vi "Get Lockstep Info.vi"(8 "error in (no error)":errorcluster, 9 "Device Number":string, 10 "Lockstep Group (1)":u8=1, 11 "VISA resource name":refnum<visa-resource-name>) -> (0 "error out":errorcluster, 1 "Axis Offsets":i32[](array[numeric]), 2 "Axis Numbers":i32[](array[numeric]), 3 "VISA resource name out":refnum<visa-resource-name>, 4 "Axis Twists":i32[](array[numeric]))   [LabVIEW 2015, in "Zaber A Series.lvlib"]
doc: "Returns information about a lockstep group. The outputs are:\n- The axis numbers of the axes in the group.\n- The position offsets of each axis relative to the first one, in microsteps.\n- The current twist of each axis relative to the first one.\n\nThis VI requires that the Initialize VI has been called with the same serial port and that the specified lockstep group has been configured."
uses:
  Zaber A Series.lvlib
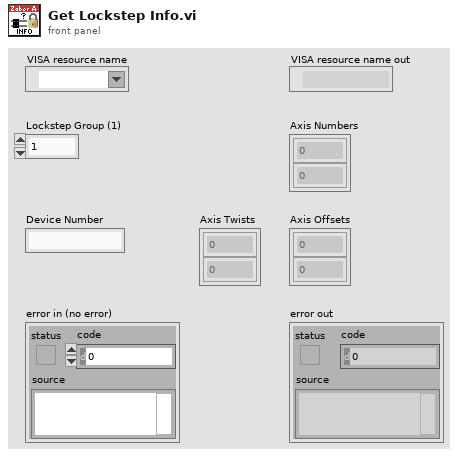
[diagram p1: front panel]
types:
  T1 = cluster{"Device":string, "Axis":string, "Reply Flag":string, "Status":string, "Warning Flags":string, "Data":string}
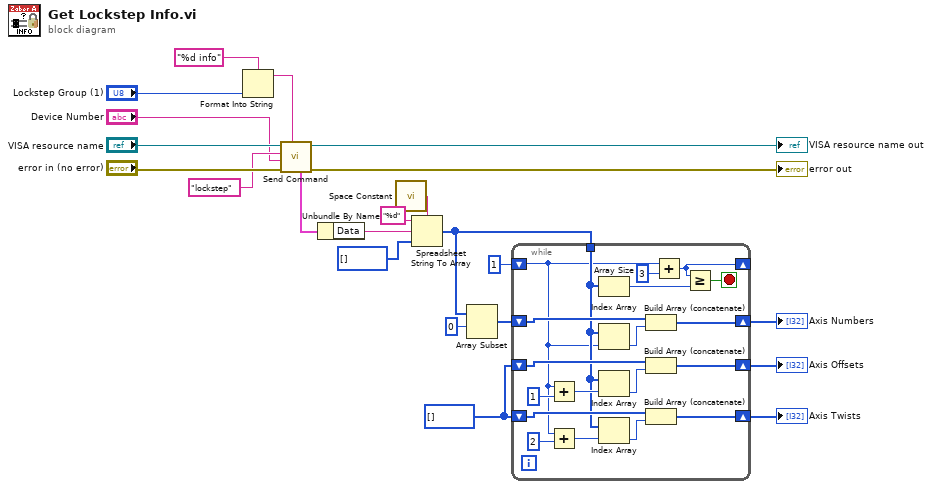
[diagram p0: block diagram]
diagram:
  w2 = i32[] [] ("Axis Offsets")
  n1 = Format Into String(format string="%d info", "Lockstep Group (1)") -> (resulting string=w10:string)  [unwired: 2 in, 1 out]
  n2 = call "Send Command.vi"("Data"=w10, "error in (no error)"="error in (no error)", "Device and Axis"="Device Number", "Command"="lockstep", "VISA resource name"="VISA resource name") -> ("error out"=→"error out":errorcluster, "VISA resource name out"=→"VISA resource name out":refnum<visa-resource-name>, "First Response Bundle"=w9:T1)  [unwired: 1 in, 3 out]
  n3 = Unbundle By Name(w9) -> ("Data"=w19:string)
  n4 = call <vilib>:"Space Constant.vi"() -> ("String"=w20:string)
  n5 = Spreadsheet String To Array(delimiter (Tab)=w20, format string="%d", spreadsheet string=w19, array type (2D Dbl)=i32[] []) -> (array=w4:i32[])
  n6 = Array Subset(array=w4, index=0) -> (w6:i32[])  [unwired: 1 in]
  n7 = while {
    shift-right: [w25] -> _
    shift-left: 1 -> [w23]
    shift-right: [w38] -> w7
    shift-left: w6 -> [w40]
    tunnel: w4 -> [w27]
    shift-right: [w34] -> w3
    shift-left: w2 -> [w35]
    shift-right: [w32] -> w1
    shift-left: w2 -> [w33]
    stop <- w24 stop-if-true
    n8 = Add(x=w23, y=1) -> (x+y=w28:i32)
    n9 = Add(x=w23, y=2) -> (x+y=w29:i32)
    n10 = Array Size(array=w27) -> (size(s)=w26:i32)
    n11 = Index Array(array=w27, index=w23) -> (element=w39:i32)
    n12 = Index Array(array=w27, index=w28) -> (element=w37:i32)
    n13 = Index Array(array=w27, index=w29) -> (element=w36:i32)
    n14 = Build Array (concatenate)(w40, w39) -> (w38:i32[])
    n15 = Build Array (concatenate)(w35, w37) -> (w34:i32[])
    n16 = Build Array (concatenate)(w33, w36) -> (w32:i32[])
    n17 = Add(x=w23, y=3) -> (x+y=w25:i32)
    n18 = Greater Or Equal?(x=w25, y=w26) -> (x >= y?=w24:bool)
  }
  "Axis Numbers" <- w7
  "Axis Offsets" <- w3
  "Axis Twists" <- w1
